vi "Serial_readV3_single.vi"() -> ()   [LabVIEW 2014]
uses:
  <vilib>/Instr/_visa.llb/VISA Set IO Buffer Mask.ctl
  <vilib>/Instr/_visa.llb/VISA Flush IO Buffer Mask.ctl
  <vilib>/Instr/_visa.llb/VISA Configure Serial Port (Instr).vi
panel:
  out "Sensor1":i32[](graph)=[3, 2, 3, 3, 3, 0, 4, 5, 1, 1, 4, 2, 2, 1, 0, 4, 2, 2, 0, 1, 2, 3, 1, 3, 4, 1, 1, 4, 3, 0, 3, 2, 4, 3, 3, 1, 2, 2, 3, 2, 1, 3, 4, 3, 1, 3, 0, 4, 4, 2, 2, 0, 2, 4, 4, 2, 3, 2, 2, 4, 2, 0, 4, 4, 2, 2, 2, 2, 2, 2, 1, 4, 0, 1, 3, 3, 1, 3, 4, 2, 1, 3, 4, 2, 2, 3, 2, 0, 4, 4, 3, 3, 1, 2, 4, 4, 4, 0, 2, 17, 2, 4, 2, 3, 2, 3, 2, 2, 4, 4, 3, 4, 1, 0, 1, 0, 3, 4, 4, 3, 0, 3, 2, 3, 5, 1, 0, 2, 1, 0, 3, 2, 1, 3, 2, 4, 2, 0, 0, 2, 2, 2, 1, 0, 4, 1, 4, 1, 4, 3, 2, 1, 2, 4, 0, 29, 2, 1, 2, 2, 8, 1, 3, 4, 2, 2, 13, 2, 1, 0, 1, 1, 4, 3, 2, 4, 2, 1, 4, 5, 1, 4, 3, 1, 0, 2, 1, 4, 3, 0, 2, 4, 2, 2, 4, 2, 1, 2, 3, 3, 11, 1, 4, 4, 2, 4, 2, 3, 1, 1, 2, 3, 3, 4, 3, 0, 1, 2, 2, 5, 21, 4, 1, 2, 4, 2, 1, 3, 2, 3, 3, 0, 4, 3, 1, 3, 1, 4, 1, 3, 1, 5, 1, 4, 1, 3, 0, 3, 5, 3, 2, 2, 1, 4, 3, 2, 2, 4, 2, 3, 2, 1, 0, 1, 0, 3, 4, 6, 0, 4, 2, 2, 4, 2, 4, 4, 4, 2, 2, 1, 4, 2, 3, 3, 4, 4, 2, 0, 0, 0, 1, 3, 3, 2, 3, 1, 3, 2, 1, 1, 4, 6, 4, 1, 2, 10, 3, 4, 2, 3, 3, 3, 1, 3, 1, 3, 2, 4, 1, 4, 0, 2, 1, 4, 0, 0, 1, 3, 3, 4, 4, 0, 4, 3, 3, 8, 0, 2, 3, 1, 2, 1, 2, 4, 1, 3, 7, 4, 1, 3, 0, 1, 2, 3, 2, 1, 4, 4, 3, 4, 2, 4, 2, 4, 4, 1, 1, 1, 0, 4, 4, 1, 2, 4, 7, 4, 0, 1, 4, 1, 0, 11, 3, 3, 4, 2, 5, 4, 3, 4, 1, 5, 3, 3, 4, 1, 9, 4, 1, 2, 1, 4, 4, 3, 4, 1, 4, 2, 4, 4, 2, 2, 1, 2, 0, 1, 0, 5, 4, 2, 4, 3, 3, 4, 0, 3, 1, 2, 2, 5, 1, 4, 0, 0, 5, 3, 2, 3, 4, 5, 0, 2, 1, 2, 0, 2, 2, 4, 1, 4, 4, 3, 3, 2, 2, 6, 4, 3, 3, 3, 2, 3, 2, 4, 4, 2, 2, 4, 4, 2, 0, 1, 4, 1, 2, 3, 5, 1, 3, 1, 3, 1, 4, 4, 1, 4, 3, 2, 3, 2, 3, 2, 4, 2, 1, 4, 4, 3, 5, 1, 0, 0, 5, 13, 1, 4, 2, 2, 3, 4, 1, 4, 1, 1, 2, 1, 3, 2, 3, 4, 3, 3, 4, 1, 2, 4, 2, 3, 2, 2, 4, 5, 1, 1, 1, 4, 13, 1, 1, 1, 4, 1, 0, 2, 1, 1, 4, 2, 3, 0, 0, 0, 1, 0, 4, 0, 0, 0, 0, 0, 0, 0, 2, 0, 0, 3, 1, 1, 2, 0, 2, 2, 1, 2, 0, 3, 1, 2, 2, 1, 2, 3, 1, 4, 0, 4, 1, 2, 2, 4, 1, 2, 0, 4, 1, 3, 2, 3, 0, 3, 3, 2, 4, 4, 4, 4, 3, 2, 9, 4, 1, 0, 1, 4, 4, 1, 3, 4, 3, 0, 3, 5, 0, 3, 2, 0, 4, 2, 4, 1, 1, 4, 4, 2, 4, 4, 2, 3, 3, 3, 4, 0, 1, 2, 3, 3, 3, 2, 2, 4, 3, 3, 1, 8, 1, 0, 4, 4, 4, 0, 2, 4, 4, 0, 1, 3, 4, 1, 4, 3, 2, 3, 4, 5, 0, 3, 4, 3, 3, 4, 2, 1, 2, 2, 4, 2, 4, 3, 1, 0, 2, 4, 3, 4, 1, 4, 3, 3, 2, 4, 1, 3, 4, 1, 1, 3, 2, 3, 4, 1, 0, 4, 4, 2, 1, 3, 3, 3, 4, 3, 4, 1, 4, 1, 4, 4, 3, 0, 2, 2, 2, 1, 2, 0, 1, 2, 0, 4, 2, 6, 3, 2, 4, 5, 4, 1, 4, 3, 4, 2, 4, 3, 3, 3, 1, 4, 3, 2, 4, 2, 1, 4, 2, 3, 1, 4, 1, 2, 1, 1, 1, 4, 0, 2, 2, 1, 4, 4, 2, 2, 0, 2, 3, 3, 2, 4, 1, 3, 0, 3, 3, 4, 3, 2, 3, 2, 4, 2, 4, 3, 0, 4, 0, 3, 4, 1, 4, 1, 1, 0, 3, 3, 1, 4, 4, 3, 4, 5, 0, 2, 3, 4, 2, 3, 4, 3, 5, 3, 1, 4, 2, 4, 1, 1, 0, 3, 3, 2, 2, 4, 2, 4, 2, 4, 3, 4, 1, 1, 2, 4, 3, 3, 3, 2, 1, 3, 3, 4, 4, 4, 4, 5, 1, 4, 2, 1, 2, 4, 4, 1, 3, 2, 3, 2, 4, 0, 3, 2, 1, 0, 2, 0, 4, 1, 2, 4, 0, 3, 1, 5, 0, 3, 1, 2, 4, 4, 2, 1, 1, 4, 2, 0, 2, 3, 1, 4, 5, 3, 4, 2, 1, 0, 1, 1, 4, 0, 0, 4, 1, 3, 4, 4, 7, 0, 1, 2, 0, 2, 4, 4, 2, 3, 3, 2, 3, 2, 1, 3, 0, 2, 4, 2, 2, 5, 1, 4, 3, 2, 2, 2, 3, 2, 1, 2, 2, 3, 2, 5, 2, 3, 3, 2, 4, 2, 4, 8, 4, 2, 4, 4, 0, 4, 2, 4, 1, 4, 1, 4, 2, 4, 4, 2, 5, 3, 9, 1, 3, 3, 2, 4, 8, 2, 4, 4, 3, 2, 5, 1, 1, 2, 4, 3, 4, 4, 2, 3, 4, 3, 4, 1, 2, 4, 1, 2, 1, 0, 4, 2, 7, 4, 4, 4, 2, 1, 3, 2, 2, 2, 6, 4, 0, 2, 4, 2, 4, 4, 4, 3, 4, 0, 16, 1, 4, 5, 3, 2, 1, 4, 1, 1, 0, 3, 4, 3, 1, 4, 3, 2, 2, 1, 4, 2, 1, 3, 2, 3, 1, 4, 3, 1, 4, 0, 3, 2, 2, 3, 5, 4, 0, 4, 1, 3, 1, 4, 1, 2, 4, 17, 4, 1, 4, 3, 4, 2, 1, 4, 4, 4, 5, 4, 4, 4, 1, 4, 6, 2, 8, 3, 1, 3, 4, 4, 4, 2, 1, 2, 3, 0, 0, 3, 4, 4, 4, 4, 5, 3, 1, 4]
  in  "milliseconds to wait":u32=500
  in  "stop":bool
  in  "VISA resource name":refnum<visa-resource-name>
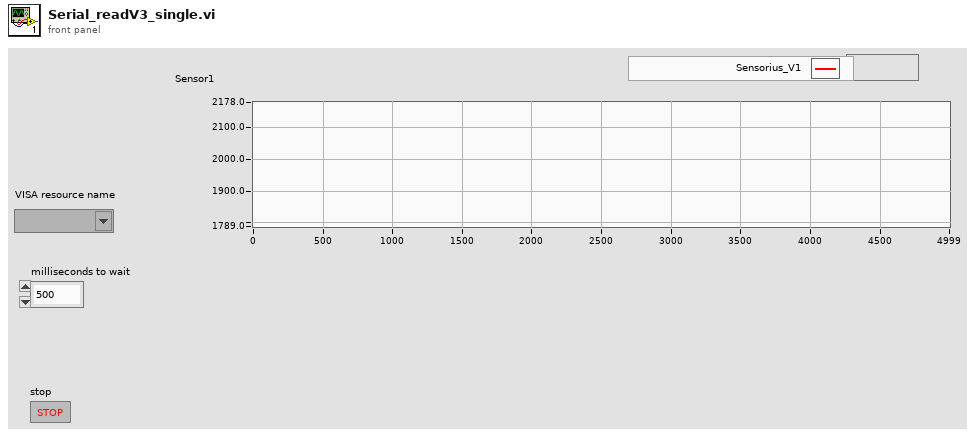
[diagram p1: front panel]
types:
  T1 = typedef "VISA Set IO Buffer Mask.ctl" = u16
  T2 = typedef "VISA Flush IO Buffer Mask.ctl" = u16
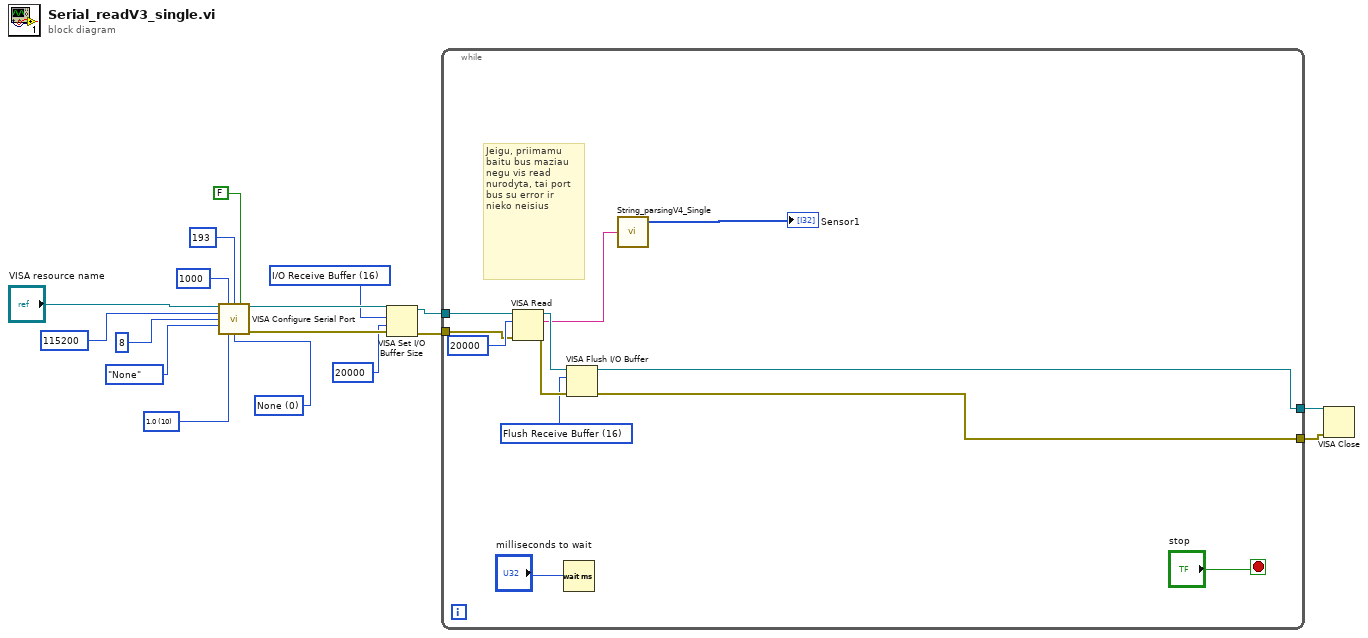
[diagram p0: block diagram]
diagram:
  w7 = T1 16 items=["I/O Receive Buffer"=16, "I/O Transmit Buffer"=32, "I/O Receive and Transmit Buffer"=48] ("Mask")
  w13 = u16 0 items=["None", "XON/XOFF", "RTS/CTS", "XON/XOFF & RTS/CTS", "DTR/DSR", "XON/XOFF & DTR/DSR"] ("flow control (0:none)")
  w14 = u16 10 items=["1.0"=10, "1.5"=15, "2.0"=20] ("stop bits (10: 1 bit)")
  n1 = call-poly "VISA Configure Serial Port"("VISA resource name"="VISA resource name", "timeout (10sec)"=u32 1000, "termination char\n(0xA = '\\n' = LF)"=u8 193 ("termination char\n(0xA = '\\n' = LF)"), "Enable Termination\nChar (T)"=FALSE ("Enable Termination\nChar (T)"), "baud rate (9600)"=u32 115200, "data bits (8)"=u16 8, "parity (0:none)"=enum16{"None", "Odd", "Even", "Mark", "Space"}."None", "stop bits (10: 1 bit)"=w14, "flow control (0:none)"=w13) -> ("VISA resource name out"=w9:refnum<visa-resource-name>, "error out"=w10:errorcluster)  [unwired: 5 in]
  n2 = VISA Set I/O Buffer Size(VISA resource name=w9, mask (16)=w7, size (4096)=u32 20000, error in (no error)=w10) -> (VISA resource name out=w3:refnum<visa-resource-name>, error out=w6:errorcluster)
  n3 = while {
    tunnel: w3 -> [w29]
    tunnel: w6 -> [w26]
    tunnel: [w20] -> w2
    tunnel: [w19] -> w1
    stop <- "stop" stop-if-true
    w23 = T2 16 items=["Flush Receive Buffer"=16, "Write Transmit Buffer to Device"=32, "Flush Receive Buffer (No I/O)"=64, "Flush Transmit Buffer"=128] ("Mask")
    # "Jeigu, priimamu baitu bus maziau negu vis read nurodyta, tai port bus su error ir nieko neisius"
    n4 = VISA Read(VISA resource name=w29, byte count=u32 20000, error in (no error)=w26) -> (VISA resource name out=w25:refnum<visa-resource-name>, read buffer=w21:string, error out=w24:errorcluster)  [unwired: 1 out]
    n5 = Wait (ms)(milliseconds to wait="milliseconds to wait") -> ()  [unwired: 1 out]
    n6 = VISA Flush I/O Buffer(VISA resource name=w25, mask (16)=w23, error in (no error)=w24) -> (VISA resource name out=w20:refnum<visa-resource-name>, error out=w19:errorcluster)
    n7 = call "String_parsingV4_Single.vi"("input string"=w21) -> ("V1"=→"Sensor1":i32[])  [unwired: 4 in]
  }
  n8 = VISA Close(VISA resource name=w2, error in (no error)=w1) -> ()  [unwired: 1 out]
